vi "XY go when press start.vi"() -> ()   [LabVIEW 2016]
uses:
  Classes/Controllers/Motion/Copy of A3200 Folder/A3200.lvclass
panel:
  in  "stop":bool
  in  "start":bool
  out "XYZTheta Out":dbl[](array[numeric])
  in  "Speed":dbl
  in  "XY":dbl[](array[numeric])
  out "XYZTheta Out 2":dbl[](array[numeric])
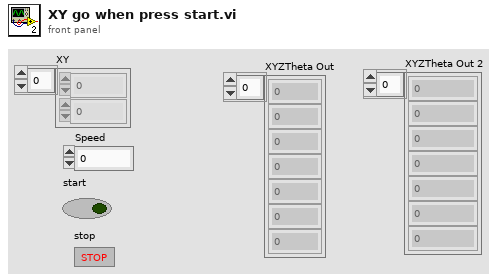
[diagram p1: front panel]
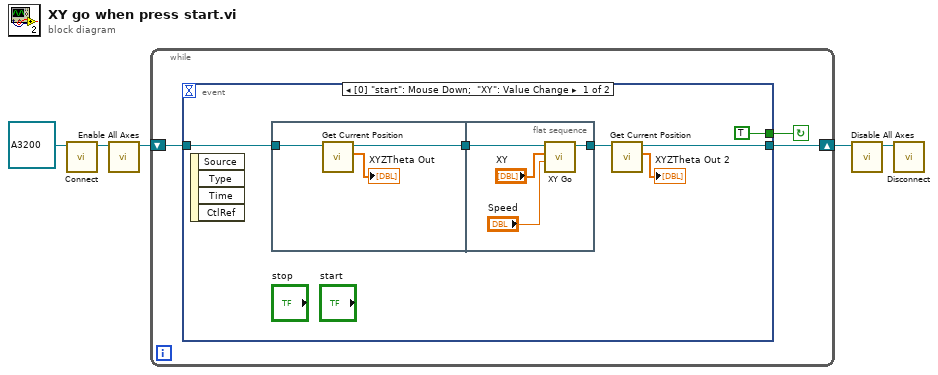
[diagram p0: block diagram]
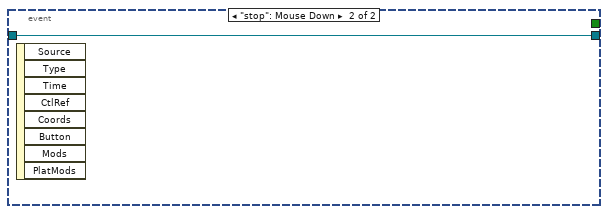
[diagram p2: hidden frame]
diagram:
  n1 = call-dynamic "Connect.vi"("Gantry in"=refnum<class "A3200.lvclass"> refnum ("Copy of A3200.lvclass")) -> ("Gantry out"=w4:refnum<class "A3200.lvclass">)  [unwired: 9 in, 1 out]
  n2 = call-dynamic "Enable All Axes.vi"("A3200 in"=w4) -> ("A3200 out"=w3:refnum<class "A3200.lvclass">)  [unwired: 9 in, 1 out]
  n3 = while {
    shift-right: [w8] -> w2
    shift-left: w3 -> [w7]
    stop <- w6 continue-if-true
    n4 = event shown="[0] \"start\": Mouse Down;  \"XY\": Value Change" {
      selector: _ -> [_ _]
      dyn-events: _ -> [_ _]
      timeout: _ -> [_ _]
      tunnel: [w12 w22] -> w8
      tunnel: w7 -> [w13 w22]
      tunnel: [TRUE _] -> w6
      event "start": Mouse Down; "XY": Value Change {
        n5 = event-data() -> ()  [unwired: 1 in, 4 out]
        n6 = flat-sequence {
          tunnel: w13 -> [w17]
          tunnel: [w16] -> w10
          tunnel: w10 -> [w21]
          tunnel: [w18] -> w9
          frame #0 {
            n7 = call-dynamic "Get Current Position.vi"("Gantry in"=w17) -> ("XYZTheta Out"=→"XYZTheta Out":dbl[], "Gantry out"=w16:refnum<class "A3200.lvclass">)  [unwired: 8 in, 1 out]
          }
          frame #1 {
            n8 = call-dynamic "XY Go.vi"("Speed"="Speed", "XY"="XY", "Gantry in"=w21) -> ("Gantry out"=w18:refnum<class "A3200.lvclass">)  [unwired: 7 in, 1 out]
          }
        }
        n9 = call-dynamic "Get Current Position.vi"("Gantry in"=w9) -> ("XYZTheta Out"=→"XYZTheta Out 2":dbl[], "Gantry out"=w12:refnum<class "A3200.lvclass">)  [unwired: 8 in, 1 out]
      }
      event "stop": Mouse Down {
        n10 = event-data() -> ()  [unwired: 1 in, 8 out]
      }
    }
  }
  n11 = call-dynamic "Disable All Axes.vi"("Gantry in"=w2) -> ("Gantry out"=w1:refnum<class "A3200.lvclass">)  [unwired: 9 in, 1 out]
  n12 = call-dynamic "Disconnect.vi"("Gantry in"=w1) -> ()  [unwired: 9 in, 1 out]
